vi "Three Register Calculation.VI"(1 "operation":i32, 2 "before last":dbl format="%0.2f", 3 "last":dbl format="%0.2f") -> (0 "result":dbl format="%0.2f")   [LabVIEW 2014, in "NI_Gmath.lvlib"]
uses:
  NI_Gmath.lvlib
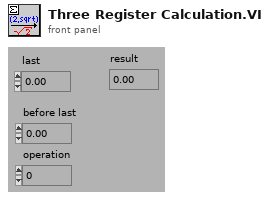
[diagram p1: front panel]
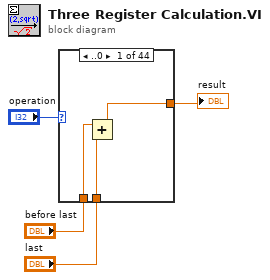
[diagram p0: block diagram]
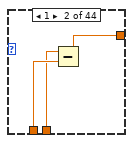
[diagram p2: hidden frame]
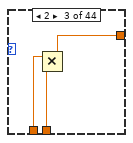
[diagram p3: hidden frame]
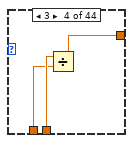
[diagram p4: hidden frame]
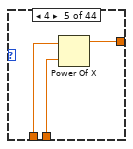
[diagram p5: hidden frame]
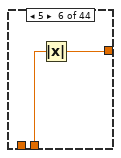
[diagram p6: hidden frame]
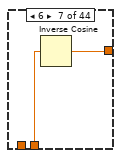
[diagram p7: hidden frame]
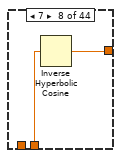
[diagram p8: hidden frame]
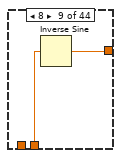
[diagram p9: hidden frame]
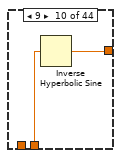
[diagram p10: hidden frame]
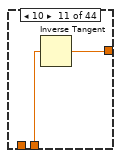
[diagram p11: hidden frame]
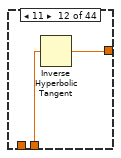
[diagram p12: hidden frame]
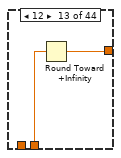
[diagram p13: hidden frame]
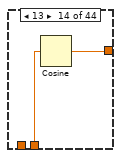
[diagram p14: hidden frame]
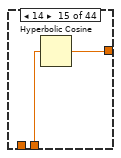
[diagram p15: hidden frame]
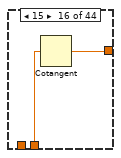
[diagram p16: hidden frame]
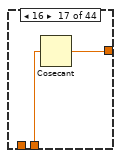
[diagram p17: hidden frame]
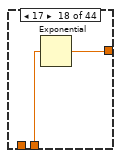
[diagram p18: hidden frame]
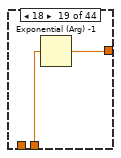
[diagram p19: hidden frame]
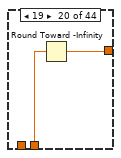
[diagram p20: hidden frame]
diagram:
  n1 = case shown="..0" "operation" {
    tunnel: "before last" -> [w7 w9 w13 w14 w17 _ _ _ _ _ _ _ _ _ _ _ _ _ _ _ _ _ _ _ _ _ _ _ _ _ _ _ _ _ _ _ _ _ _ _ _ _ _ _]
    tunnel: "last" -> [w6 w8 w12 w15 w18 w21 w23 w25 w27 w29 w31 w33 w35 w37 w39 w41 w43 w45 w47 w49 w51 w53 w55 w56 w64 w67 w69 w71 _ w73 w75 w77 w79 w81 w83 w85 w87 w89 w93 w95 w97 w99 w101 w103]
    tunnel: [w5 w10 w11 w16 w19 w20 w22 w24 w26 w28 w30 w32 w34 w36 w38 w40 w42 w44 w46 w48 w50 w52 w54 w57 w63 w66 w68 w70 w72 w74 w76 w78 w80 w82 w84 w86 w88 w90 w91 w94 w96 w98 w100 w102] -> w2
    frame ..0 {
      n2 = Add(x=w7, y=w6) -> (x+y=w5:dbl)
    }
    frame 1 {
      n3 = Subtract(x=w8, y=w9) -> (x-y=w10:dbl)
    }
    frame 2 {
      n4 = Multiply(x=w13, y=w12) -> (x*y=w11:dbl)
    }
    frame 3 {
      n5 = Divide(x=w15, y=w14) -> (x/y=w16:dbl)
    }
    frame 4 {
      n6 = Power Of X(1:w18, 2:w17) -> (0:w19:dbl)
    }
    frame 5 {
      n7 = Absolute Value(x=w21) -> (abs(x)=w20:dbl)
    }
    frame 6 {
      n8 = Inverse Cosine(1:w23) -> (0:w22:dbl)
    }
    frame 7 {
      n9 = Inverse Hyperbolic Cosine(1:w25) -> (0:w24:dbl)
    }
    frame 8 {
      n10 = Inverse Sine(1:w27) -> (0:w26:dbl)
    }
    frame 9 {
      n11 = Inverse Hyperbolic Sine(1:w29) -> (0:w28:dbl)
    }
    frame 10 {
      n12 = Inverse Tangent(1:w31) -> (0:w30:dbl)
    }
    frame 11 {
      n13 = Inverse Hyperbolic Tangent(1:w33) -> (0:w32:dbl)
    }
    frame 12 {
      n14 = Round Toward +Infinity(x=w35) -> (ceil(x): smallest int >= x=w34:dbl)
    }
    frame 13 {
      n15 = Cosine(x=w37) -> (cos(x)=w36:dbl)
    }
    frame 14 {
      n16 = Hyperbolic Cosine(1:w39) -> (0:w38:dbl)
    }
    frame 15 {
      n17 = Cotangent(1:w41) -> (0:w40:dbl)
    }
    frame 16 {
      n18 = Cosecant(1:w43) -> (0:w42:dbl)
    }
    frame 17 {
      n19 = Exponential(1:w45) -> (0:w44:dbl)
    }
    frame 18 {
      n20 = Exponential (Arg) -1(1:w47) -> (0:w46:dbl)
    }
    frame 19 {
      n21 = Round Toward -Infinity(1:w49) -> (0:w48:dbl)
    }
    frame 20 {
      n22 = Mantissa & Exponent(0:w51) -> (2:w50:dbl)  [unwired: 1 out]
    }
    frame 21 {
      n23 = Mantissa & Exponent(0:w53) -> (1:w52:dbl)  [unwired: 1 out]
    }
    frame 22 {
      n24 = Round Toward -Infinity(1:w55) -> (0:w54:dbl)
    }
    frame 23 {
      n25 = Greater Or Equal To 0?(x=w56) -> (x >= 0?=w58:bool)
      n26 = case shown="False" w58 {
        tunnel: w56 -> [w60 w62]
        tunnel: [w59 w61] -> w57
        frame False {
          n27 = Round Toward +Infinity(x=w60) -> (ceil(x): smallest int >= x=w59:dbl)
        }
        frame True {
          n28 = Round Toward -Infinity(1:w62) -> (0:w61:dbl)
        }
      }
    }
    frame 24 {
      n29 = Natural Logarithm(1:w64) -> (0:w63:dbl)
    }
    frame 25 {
      n30 = Increment(x=w67) -> (x+1=w65:dbl)
      n31 = Natural Logarithm(1:w65) -> (0:w66:dbl)
    }
    frame 26 {
      n32 = Logarithm Base 10(1:w69) -> (0:w68:dbl)
    }
    frame 27 {
      n33 = Logarithm Base 2(1:w71) -> (0:w70:dbl)
    }
    frame 28 {
      n34 = Random Number (0-1)() -> (number: 0 to 1=w72:dbl)
    }
    frame 29 {
      n35 = Secant(1:w73) -> (0:w74:dbl)
    }
    frame 30 {
      n36 = Sign(1:w75) -> (0:w76:dbl)
    }
    frame 31 {
      n37 = Sine(x=w77) -> (sin(x)=w78:dbl)
    }
    frame 32 {
      n38 = Sinc(1:w79) -> (0:w80:dbl)
    }
    frame 33 {
      n39 = Hyperbolic Sine(1:w81) -> (0:w82:dbl)
    }
    frame 34 {
      n40 = Square Root(x=w83) -> (sqrt(x)=w84:dbl)
    }
    frame 35 {
      n41 = Tangent(1:w85) -> (0:w86:dbl)
    }
    frame 36 {
      n42 = Hyperbolic Tangent(1:w87) -> (0:w88:dbl)
    }
    frame 37 {
      n43 = call "(Incomplete) Gamma Function (obs).vi"("x"=w89) -> ("g(x, a)"=w90:dbl)  [unwired: 2 in]
    }
    frame 38 {
      n44 = Multiply(x=3.141592653589793, y=w93) -> (x*y=w91:dbl)
    }
    frame 39 {
      n45 = call "Cosine Integral.vi"("x"=w95) -> ("Ci(x)"=w94:dbl)  [unwired: 2 in]
    }
    frame 40 {
      n46 = call "Sine Integral.vi"("x"=w97) -> ("Si(x)"=w96:dbl)  [unwired: 2 in]
    }
    frame 41 {
      n47 = call "Spike Function.vi"("x"=w99) -> ("spike(x)"=w98:dbl)
    }
    frame 42 {
      n48 = call "Step Function.vi"("x"=w101) -> ("step(x)"=w100:dbl)
    }
    frame 43.. {
      n49 = call "Square Function.vi"("x"=w103) -> ("square(x)"=w102:dbl)
    }
  }
  "result" <- w2
